vi "meth.Table2NamedCluster.vi"(0 "class.GLue in":refnum<class "class.GLue.lvclass">, 7 "Names":string[](array[string]), 11 "error in":errorcluster) -> (4 "class.GLue out":refnum<class "class.GLue.lvclass">, 8 "Cluster":variant, 15 "error out":errorcluster)   [LabVIEW 2014, in "GLue.lvlib" / "class.GLue.lvclass"]
uses:
  class.GLue.lvclass
  class.GLue.lvclass/class.GLue.ctl
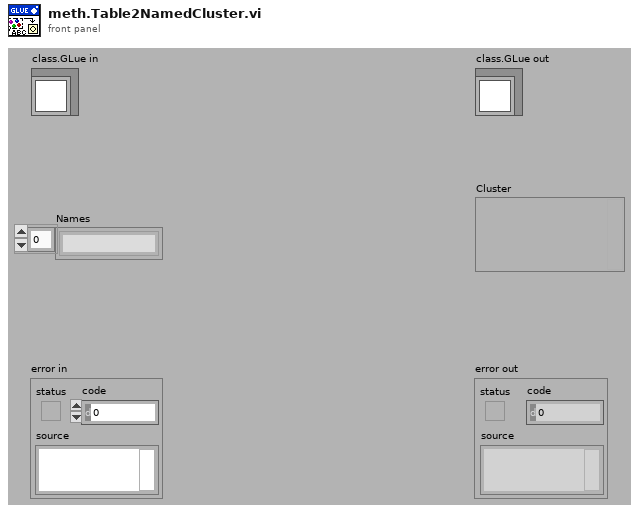
[diagram p1: front panel]
types:
  T1 = typedef "GLue.lvlib/class.GLue.lvclass/typedef.Types.ctl" = enum16{"Nil", "Bool", "LightUserData", "Number", "String", "Table", "Function", "UserData", "Thread"}
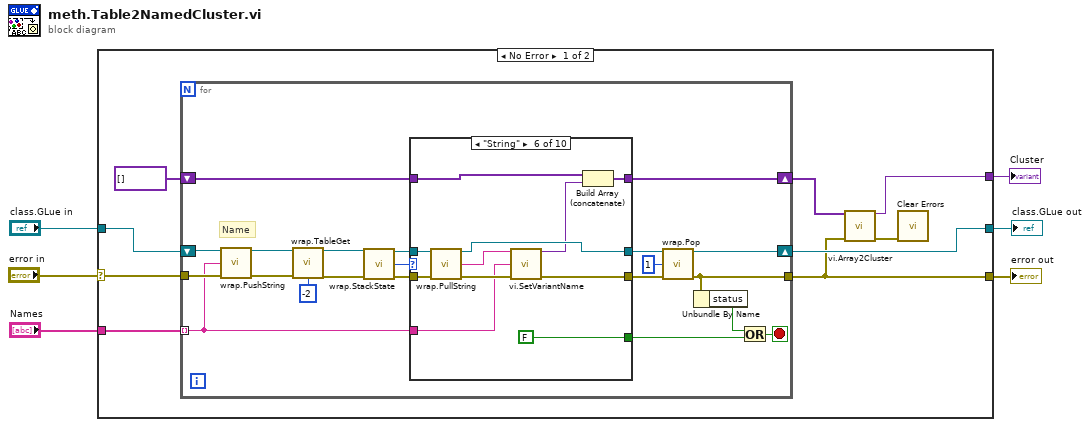
[diagram p0: block diagram]
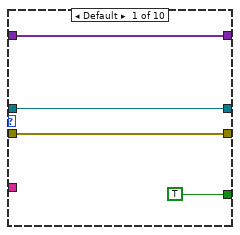
[diagram p2: hidden frame]
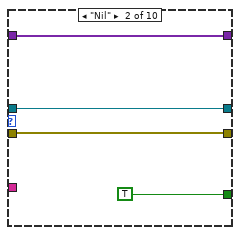
[diagram p3: hidden frame]
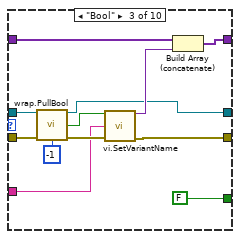
[diagram p4: hidden frame]
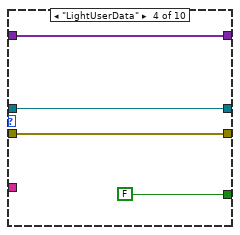
[diagram p5: hidden frame]
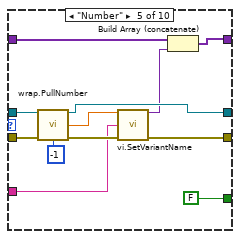
[diagram p6: hidden frame]
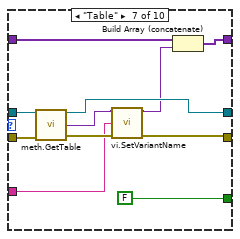
[diagram p7: hidden frame]
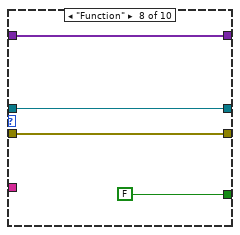
[diagram p8: hidden frame]
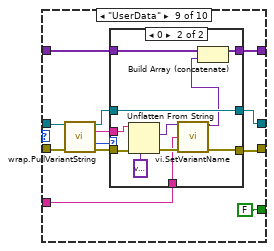
[diagram p9: hidden frame]
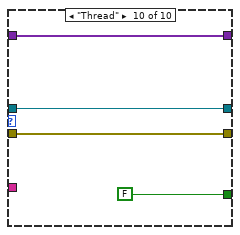
[diagram p11: hidden frame]
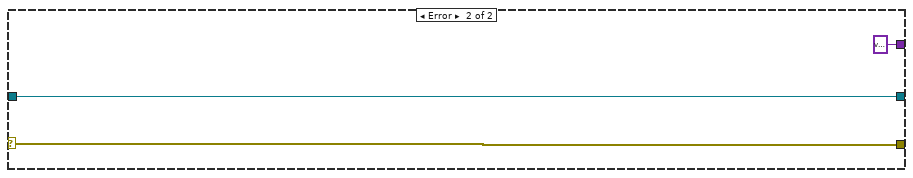
[diagram p12: hidden frame]
diagram:
  n1 = case shown="No Error" "error in" {
    selector: "error in" -> [w7 w131]
    tunnel: [w10 w131] -> w5
    tunnel: [w11 w130] -> w3
    tunnel: "class.GLue in" -> [w8 w130]
    tunnel: [w12 variant ("Cluster")] -> w2
    tunnel: "Names" -> [w9 _]
    frame No Error {
      n2 = for {
        tunnel: w7 -> [w24]
        shift-right: [w33] -> w14
        shift-left: variant[] [] ("Table") -> [w36]
        shift-right: [w35] -> w11
        shift-left: w8 -> [w23]
        tunnel: [w34] -> w10
        tunnel: w9 -> [w16] mode=indexing
        stop <- w17 stop-if-true
        # "Name"
        n3 = call "wrap.PushString.vi"("class.GLue in"=w23, "String"=w16, "error in (no error)"=w24) -> ("class.GLue out"=w21:refnum<class "class.GLue.lvclass">, "error out"=w22:errorcluster)  [unwired: 11 in]
        n4 = call "wrap.TableGet.vi"("class.GLue in"=w21, "error in (no error)"=w22, "Index"=-2) -> ("class.GLue out"=w20:refnum<class "class.GLue.lvclass">, "error out"=w19:errorcluster)  [unwired: 11 in]
        n5 = call "wrap.StackState.vi"("class.GLue in"=w20, "error in (no error)"=w19) -> ("class.GLue out"=w31:refnum<class "class.GLue.lvclass">, "TopType"=w32:T1, "error out"=w30:errorcluster)  [unwired: 10 in, 1 out]
        n6 = case shown="\"String\"" w32 {
          tunnel: w31 -> [w39 w44 w56 w59 w70 w83 w94 w97 w108 w127]
          tunnel: w30 -> [w40 w41 w55 w58 w69 w82 w93 w96 w109 w126]
          tunnel: w36 -> [w38 w42 w53 w60 w72 w81 w92 w98 w101 w128]
          tunnel: [w40 w41 w48 w58 w64 w76 w87 w96 w103 w126] -> w29
          tunnel: [w39 w44 w45 w59 w66 w78 w89 w97 w104 w127] -> w28
          tunnel: [w38 w42 w52 w60 w71 w80 w91 w98 w100 w128] -> w33
          tunnel: [TRUE TRUE FALSE FALSE FALSE FALSE FALSE FALSE FALSE FALSE] -> w25
          tunnel: w16 -> [_ _ w49 _ w63 w75 w85 _ w99 _]
          frame Default {
          }
          frame "Nil" {
          }
          frame "Bool" {
            n7 = call "wrap.PullBool.vi"("class.GLue in"=w56, "error in (no error)"=w55, "Index"=-1) -> ("class.GLue out"=w45:refnum<class "class.GLue.lvclass">, "Boolean"=w47:bool, "error out"=w50:errorcluster)  [unwired: 10 in]
            n8 = call "vi.SetVariantName.vi"("Variant in"=w47, "Name"=w49, "error in"=w50) -> ("Named Variant"=w46:variant, "error out"=w48:errorcluster)  [unwired: 11 in]
            n9 = Build Array (concatenate)(w53, w46) -> (w52:variant[])
          }
          frame "LightUserData" {
          }
          frame "Number" {
            n10 = call "wrap.PullNumber.vi"("class.GLue in"=w70, "error in (no error)"=w69, "Index"=-1) -> ("class.GLue out"=w66:refnum<class "class.GLue.lvclass">, "Number"=w62:dbl, "error out"=w65:errorcluster)  [unwired: 10 in]
            n11 = call "vi.SetVariantName.vi"("Variant in"=w62, "Name"=w63, "error in"=w65) -> ("Named Variant"=w61:variant, "error out"=w64:errorcluster)  [unwired: 11 in]
            n12 = Build Array (concatenate)(w72, w61) -> (w71:variant[])
          }
          frame "String" {
            n13 = call "wrap.PullString.vi"("class.GLue in"=w83, "error in (no error)"=w82) -> ("class.GLue out"=w78:refnum<class "class.GLue.lvclass">, "String"=w74:string, "error out"=w77:errorcluster)  [unwired: 11 in]
            n14 = call "vi.SetVariantName.vi"("Variant in"=w74, "Name"=w75, "error in"=w77) -> ("Named Variant"=w73:variant, "error out"=w76:errorcluster)  [unwired: 11 in]
            n15 = Build Array (concatenate)(w81, w73) -> (w80:variant[])
          }
          frame "Table" {
            n16 = call "meth.GetTable.vi"("class.GLue in"=w94, "error in (no error)"=w93) -> ("class.GLue out"=w89:refnum<class "class.GLue.lvclass">, "Table"=w86:variant, "error out"=w88:errorcluster)  [unwired: 11 in]
            n17 = call "vi.SetVariantName.vi"("Variant in"=w86, "Name"=w85, "error in"=w88) -> ("Named Variant"=w84:variant, "error out"=w87:errorcluster)  [unwired: 11 in]
            n18 = Build Array (concatenate)(w92, w84) -> (w91:variant[])
          }
          frame "Function" {
          }
          frame "UserData" {
            n19 = call "wrap.PullVariantString.vi"("class.GLue in"=w108, "error in (no error)"=w109) -> ("class.GLue out"=w105:refnum<class "class.GLue.lvclass">, "VarString"=w102:string, "Return"=w106:i32, "error out"=w107:errorcluster)  [unwired: 10 in]
            n20 = case shown="0" w106 {
              tunnel: w107 -> [w111 w124]
              tunnel: w105 -> [w112 w123]
              tunnel: [w112 w123] -> w104
              tunnel: [w111 w118] -> w103
              tunnel: w102 -> [_ w121]
              tunnel: w101 -> [w113 w120]
              tunnel: [w113 w119] -> w100
              tunnel: w99 -> [_ w116]
              frame Default {
              }
              frame 0 {
                n21 = Unflatten From String(type=variant ("Cluster"), binary string=w121, error in (no error)=w124) -> (value=w115:variant, error out=w117:errorcluster)  [unwired: 2 in, 1 out]
                n22 = call "vi.SetVariantName.vi"("Variant in"=w115, "Name"=w116, "error in"=w117) -> ("Named Variant"=w114:variant, "error out"=w118:errorcluster)  [unwired: 11 in]
                n23 = Build Array (concatenate)(w120, w114) -> (w119:variant[])
              }
            }
          }
          frame "Thread" {
          }
        }
        n24 = call "wrap.Pop.vi"("class.GLue in"=w28, "Num"=1, "error in (no error)"=w29) -> ("class.GLue out"=w35:refnum<class "class.GLue.lvclass">, "error out"=w34:errorcluster)  [unwired: 11 in]
        n25 = Unbundle By Name(w34) -> ("status"=w26:bool)
        n26 = Or(x=w26, y=w25) -> (x .or. y?=w17:bool)
      }
      n27 = call "vi.Array2Cluster.vi"("Array"=w14, "error in (no error)"=w10) -> ("Cluster"=w12:variant, "error out"=w15:errorcluster)  [unwired: 12 in]
      n28 = call <vilib>:"Clear Errors.vi"("error in (no error)"=w15) -> ()  [unwired: 5 in, 2 out]
    }
    frame Error {
    }
  }
  "error out" <- w5
  "class.GLue out" <- w3
  "Cluster" <- w2
